vi "URAPI_Calculator.vi"(0 "X":string="X", 3 "URAPI Script":T1={"Script"="", "Whiles"=[], "Ifs"=[], "Supress Err"=TRUE, "Errors"=""}, 4 "Formula":string="X=X+1") -> (2 "Variable Out":string, 5 "URAPI Script":T1={"Script"="", "Whiles"=[], "Ifs"=[], "Supress Err"=TRUE, "Errors"=""})   [LabVIEW 2012]
doc: "Applies a \"Formula\" to the specified variable \"X\", and returns \"Varialbe out\" as the result of this calculation."
uses:
  <userlib>/botspeak/VIs/Direct/URAPI_Control.ctl
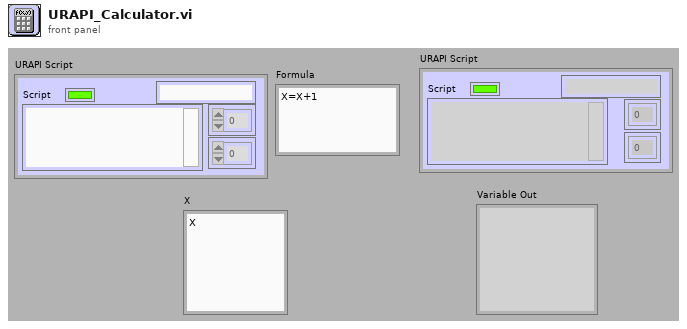
[diagram p1: front panel]
types:
  T1 = typedef "URAPI_Control.ctl" = cluster{"Script":string, "Whiles":u8[], "Ifs":u8[], "Supress Err":bool, "Errors":string}
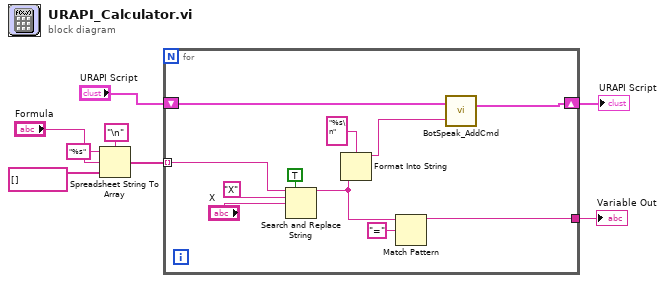
[diagram p0: block diagram]
diagram:
  n1 = Spreadsheet String To Array(delimiter (Tab)="\n", format string="%s", spreadsheet string="Formula", array type (2D Dbl)=string[] [] ("array")) -> (array=w1:string[])
  n2 = for {
    tunnel: [w14] -> w6
    shift-right: [w9] -> w7
    shift-left: "URAPI Script" -> [w11]
    tunnel: w1 -> [w12] mode=indexing
    n3 = Search and Replace String(replace all?=TRUE ("replace all? (F)"), input string=w12, search string="X" ("replace string (\"\")"), replace string="X") -> (result string=w13:string)  [unwired: 4 in, 3 out]
    n4 = Format Into String(format string="%s\n" ("string"), w13) -> (resulting string=w10:string)  [unwired: 2 in, 1 out]
    n5 = Match Pattern(string=w13, regular expression="=") -> (before substring=w14:string)  [unwired: 1 in, 3 out]
    n6 = call <userlib>:"BotSpeak_AddCmd.vi"("String"=w10, "URAPI Script"=w11) -> ("URAPI Script out"=w9:T1)  [unwired: 1 in]
  }
  "Variable Out" <- w6
  "URAPI Script" <- w7
